vi "Get package_templatemessage.vi"(8 "error in (no error)":errorcluster, 11 "gRPCid":T2) -> (0 "error out":errorcluster, 2 "package_templatemessage":T1, 3 "gRPCid out":T2)   [LabVIEW 2019, in "Service Template.lvlib"]
uses:
  Service Template.lvlib
  gRPC lv Support/Shared/grpcId.ctl
  package_templatemessage.ctl
  gRPC lv Support/Shared/TranslateGrpcError.vi
  gRPC lv Support/Server API/Server/Get Server DLL Path.vi
  <vilib>/Utility/error.llb/Error Cluster From Error Code.vi
  <vilib>/Utility/error.llb/Simple Error Handler.vi
  2f6fab4a-7742-4188-935a-b52d65d11985.vi
  gRPC lv Support/grpc-lvsupport.lvlib
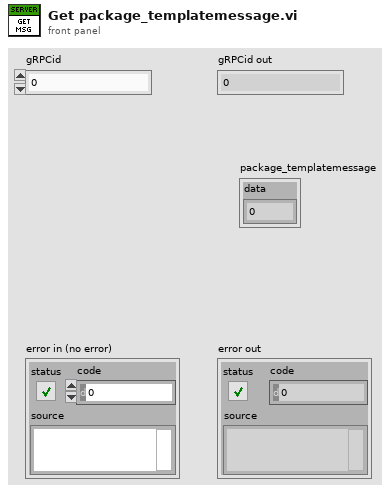
[diagram p1: front panel]
types:
  T1 = typedef "Service Template.lvlib/package_templatemessage.ctl" = cluster{"data":sgl}
  T2 = typedef "grpc-lvsupport.lvlib/grpcId.ctl" = u64
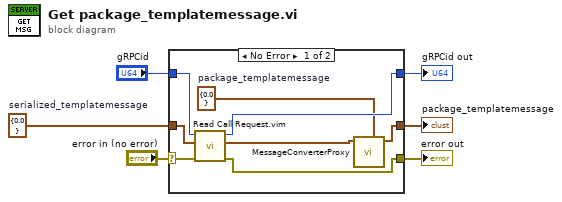
[diagram p0: block diagram]
diagram:
  w4 = T1 {"data"=0.0}  # serialized_templatemessage
  n1 = case shown="No Error" "error in (no error)" {
    selector: "error in (no error)" -> [w7 w15]
    tunnel: [w14 w16] -> w6
    tunnel: "gRPCid" -> [w13 w17]
    tunnel: w4 -> [w12 w16]
    tunnel: [w11 w17] -> w3
    tunnel: [w9 w15] -> w2
    frame No Error {
      w8 = T1 {"data"=0.0}  # package_templatemessage
      n2 = call "Read Call Request.vim"("error in"=w7, "Request Type"=w12, "gRPCid in"=w13) -> ("error out"=w9:errorcluster, "Request Data"=w10:T1, "gRPCid out"=w11:T2)  [unwired: 6 in]
      n3 = call "MessageConverterProxy.vi"("package_templatemessage_type"=w8, "example_SignalParameters_Data"=w10) -> ("package_templatemessage"=w14:T1)  [unwired: 9 in]
    }
    frame Error {
    }
  }
  "error out" <- w2
  "gRPCid out" <- w3
  "package_templatemessage" <- w6
